vi "Parse Xeryon STAT.vi"(8 "error in":errorcluster, 11 "number":i32) -> (0 "error out":errorcluster, 2 "Status":variant, 3 "STAT":string[][](table))   [LabVIEW 2019]
panel:
  in  "STAT Word":string
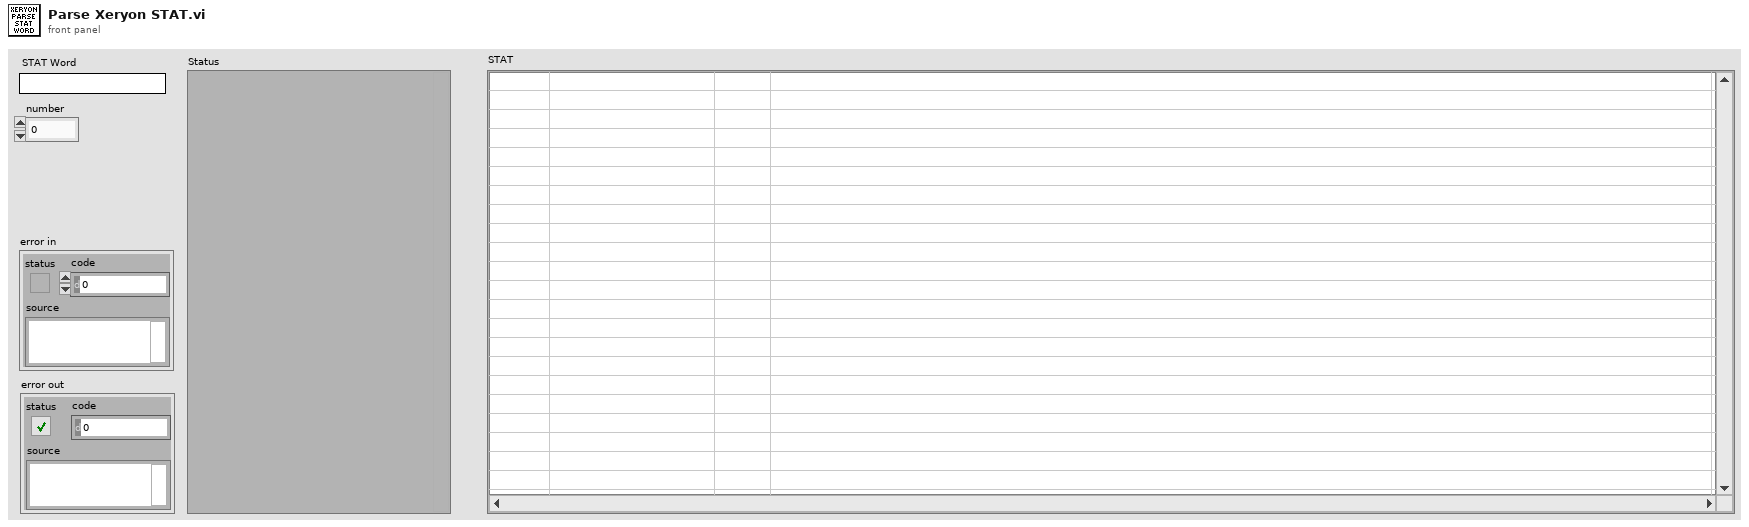
[diagram p1: front panel]
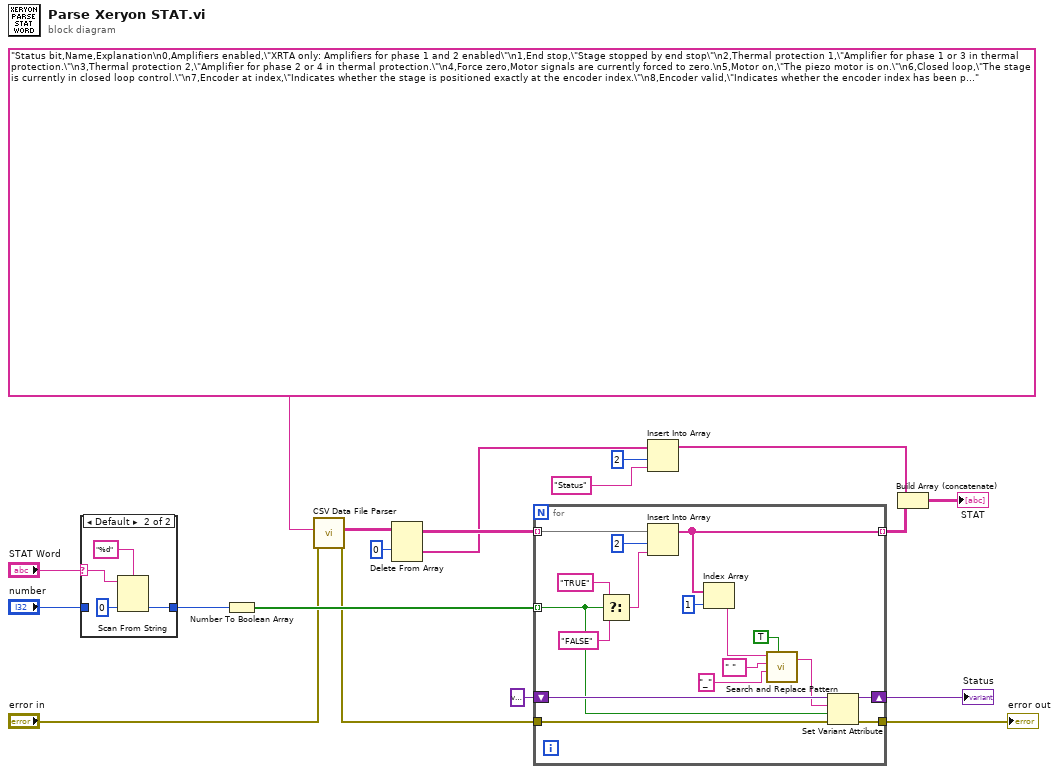
[diagram p0: block diagram]
diagram:
  n1 = case shown="Default" "STAT Word" {
    selector: "STAT Word" -> [_ w21]
    tunnel: [w20 w22] -> w7
    tunnel: "number" -> [w20 _]
    frame "" {
    }
    frame Default {
      n2 = Scan From String(format string="%d", input string=w21, default 1=0 ("default value 1")) -> (output 1=w22:i32)  [unwired: 2 in, 3 out]
    }
  }
  n3 = Number To Boolean Array(number=w7) -> (Boolean array=w15:bool[])
  n4 = call "CSV Data File Parser.vi"("error in"="error in", "CSV String"="Status bit,Name,Explanation\n0,Amplifiers enabled,\"XRTA only: Amplifiers for phase 1 and 2 enabled\"\n1,End stop,\"Stage stopped by end stop\"\n2,Thermal protection 1,\"Amplifier for phase 1 or 3 in thermal protection.\"\n3,Thermal protection 2,\"Amplifier for phase 2 or 4 in thermal protection.\"\n4,Force zero,Motor signals are currently forced to zero.\n5,Motor on,\"The piezo motor is on.\"\n6,Closed loop,\"The stage is currently in closed loop control.\"\n7,Encoder at index,\"Indicates whether the stage is positioned exactly at the encoder index.\"\n8,Encoder valid,\"Indicates whether the encoder index has been passed and therefore the encoder value reflects the absolute position, not the relative position with respect to the startup position.\"\n9,Searching index,\"Indicates whether the stage is currently searching the index position.\"\n10,Position reached,\"Indicates whether the target position is reached (within tolerance limits).\"\n11,Error compensation,\"Error compensation is on.\"\n12,Encoder error,\"Indicates an error produced by the encoder.\"\n13,Scanning,\"Indicates whether the stage is in a scanning mode.\"\n14,Left end stop,\"Indicates that the left end stop is passed.\"\n15,Right end stop,\"Indicates that the right end stop is passed.\"\n16,Error limit,\"Indicates that the position error has reached the limit set by ELIM. This can indicate a collision or mechanical limit (end of stroke).\"\n17,Searching optimal frequency,\"The driver is searching for the optimal excitation frequency of the piezo motor.\"\n18,Safety timeout triggered,\"If this is set to '1', then the safety timeout was triggered. See the explanation of the command 'TOU2' several pages back.\"\n19,EtherCAT acknowledge,\"only used when control via EtherCAT\"\n20,Emergency stop,\"not used\"\n21,Position fail,\"If this is set to '1', then the safety timeout TOU3 was triggered.\"") -> ("error out"=w4:errorcluster, "2-D Array"=w18:string[][])  [unwired: 7 in, 1 out]
  n5 = Delete From Array(array=w18, index (row)=0) -> (deleted portion=w14:string[], array with subset deleted=w16:string[][])  [unwired: 2 in]
  n6 = for {
    tunnel: w16 -> [w39] mode=indexing
    tunnel: w15 -> [w28] mode=indexing
    tunnel: [w25] -> w10 mode=indexing
    shift-right: [w34] -> w1
    shift-left: variant -> [w35]
    tunnel: w4 -> [w27]
    tunnel: [w26] -> w3
    n7 = Select(t="TRUE", s=w28, f="FALSE") -> (s? t:f=w38:string)
    n8 = Insert Into Array(array=w39, index=2, new element=w38) -> (w25:string[])
    n9 = Index Array(array=w25, index=1) -> (element=w29:string)
    n10 = call <vilib>:"Search and Replace Pattern.vi"("string"=w29, "regular expression (\"\")"=" " ("regular expression (\"\")"), "replace string (\"\")"="_" ("replace string (\"\")"), "replace all? (F)"=TRUE) -> ("result string"=w30:string)  [unwired: 1 in, 1 out]
    n11 = Set Variant Attribute(Variant=w35, name=w30, value=w28, error in=w27) -> (Variant out=w34:variant, error out=w26:errorcluster)  [unwired: 1 out]
  }
  "Status" <- w1
  "error out" <- w3
  n12 = Insert Into Array(array=w14, index=2, new element="Status" ("new element/subarray")) -> (w11:string[])
  n13 = Build Array (concatenate)(w11, w10) -> (→"STAT":string[][])
